vi "Load Values.vi"(11 "Dashboard Data":T1={"Drive PID - Low"={"D"=0.0, "F"=0.0, "RR"=0.0, "IZ"=0.0, "P"=0.0, "I"=0.0}, "Drive PID - High"={"D"=0.0, "F"=0.0, "RR"=0.0, "IZ"=0.0, "P"=0.0, "I"=0.0}, "Vision Settings"={"LED Color"={"Hue"={107.81818389892578, 139.81818389892578}, "Sat"={176.07142857142858, 255.0}, "Val"={40.53571428571429, 255.0}}, "Vision Line"=0.0, "Vision Bottom Clip"=0.0}, "Robot Name"="", "Winch Out"=0.0, "Winch In"=0.0, "Shooter Settings"={"Shooter PID"={"D"=0.0, "F"=0.0, "RR"=0.0, "IZ"=0.0, "P"=0.0, "I"=0.0}, "Instake Belt PID"={"D"=0.0, "F"=0.0, "RR"=0.0, "IZ"=0.0, "P"=0.0, "I"=0.0}, "Shooter Wheel RPM"=0.0, "Instake Belt RPM"=0.0, "Grinder Power"=0.0, "Ramp Up Speed"=0.0}} {"Vision Settings"."LED Color"."Hue" scale=0.0..255.0 scale format="%#_3g"}) -> ()   [LabVIEW 2016]
uses:
  Dashboard Data.ctl
  PID Settings.ctl
  Vision Data.ctl
  Shooter Settings.ctl
  <vilib>/Rock Robotics/WPI/Solenoid/WPI_SolenoidValue.ctl
  <vilib>/Rock Robotics/WPI/Utilities/WPI_GetSetVariantRefNum.vi
  2017 Robot Project/Ball Shooter/Implementation/Ball Shooter Global.vi
  2017 Robot Project/Winch/Implementation/Winch Globals.vi
  <vilib>/Rock Robotics/WPI/Solenoid/WPI_SolenoidSetEnum.vi
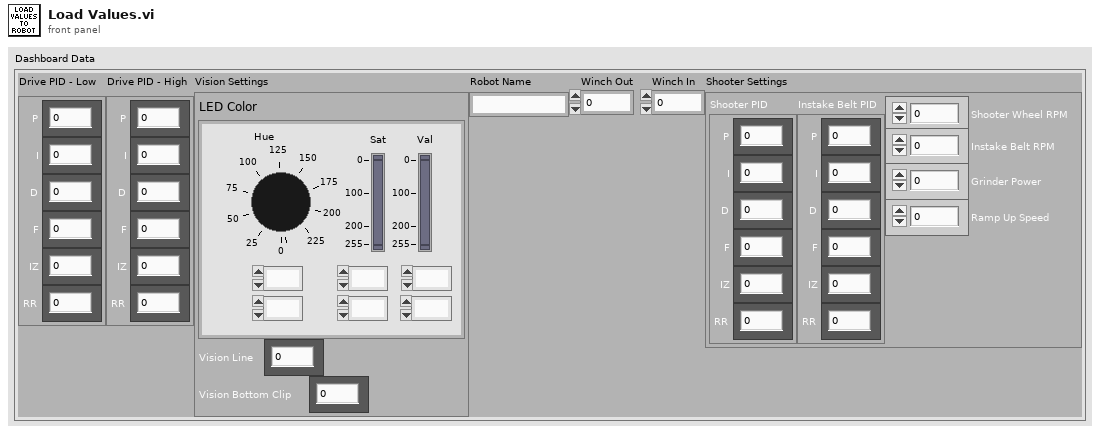
[diagram p1: front panel]
types:
  T1 = typedef "Dashboard Data.ctl" = cluster{"Drive PID - Low":T2, "Drive PID - High":T2, "Vision Settings":T3, "Robot Name":string, "Winch Out":dbl, "Winch In":dbl, "Shooter Settings":T4}
  T2 = typedef "PID Settings.ctl" = cluster{"D":dbl, "F":dbl, "RR":dbl, "IZ":dbl, "P":dbl, "I":dbl}
  T3 = typedef "Vision Data.ctl" = cluster{"LED Color":cluster{"Hue":cluster{dbl, dbl}, "Sat":cluster{dbl, dbl}, "Val":cluster{dbl, dbl}}, "Vision Line":dbl, "Vision Bottom Clip":dbl}
  T4 = typedef "Shooter Settings.ctl" = cluster{"Shooter PID":T2, "Instake Belt PID":T2, "Shooter Wheel RPM":dbl, "Instake Belt RPM":dbl, "Grinder Power":dbl, "Ramp Up Speed":dbl}
  T5 = typedef "WPI_SolenoidValue.ctl" = enum16{"Off", "On", "Forward", "Reverse"}
  T6 = typedef "WPI_RobotDriveDevRef.ctl" = cluster{"DevStatus":errorcluster, "Motors[]":T7[], "Square Inputs":bool, "Max Output":dbl}
  T7 = typedef "WPI_MotorControlDeviceRef.ctl" = cluster{"DeviceStatus":errorcluster, "Type":T8, "PWM":cluster{"PWM Channel":T9, "DeadBand":T10}, "CAN":cluster{"Device Number":u8, "SetOutput VI Ref":variant, "GetOutput VI Ref":variant, "Enable VI Ref":variant, "Disable VI Ref":variant, "Data":variant}, "Invert":bool}
  T8 = typedef "WPI_MotorControlType.ctl" = enum16{"PWM", "CAN"}
  T9 = typedef "FPGA_DIOPWMChannel.ctl" = enum8{"PWM 0", "PWM 1", "PWM 2", "PWM 3", "PWM 4", "PWM 5", "PWM 6", "PWM 7", "PWM 8", "PWM 9", "PWM MXP 0", "PWM MXP 1", "PWM MXP 2", "PWM MXP 3", "PWM MXP 4", "PWM MXP 5", "PWM MXP 6", "PWM MXP 7", "PWM MXP 8", "PWM MXP 9", "Invalid"}
  T10 = typedef "WPI_PWMDeadband.ctl" = cluster{"Name":string, "maxPositivePwm":i32, "minPositivePwm":i32, "centerPwm":i32, "maxNegativePwm":i32, "minNegativePwm":i32, "angularRange":u16}
  T11 = typedef "WPI_SolenoidDevRef.ctl" = cluster{"DevStatus":errorcluster, "Pneumatics Control Module":u8, "Forward Solenoid Channel":T12, "Reverse Solenoid Channel":T12}
  T12 = typedef "WPI_SolenoidChannel.ctl" = enum8{"Solenoid 0", "Solenoid 1", "Solenoid 2", "Solenoid 3", "Solenoid 4", "Solenoid 5", "Solenoid 6", "Solenoid 7", "Invalid"}
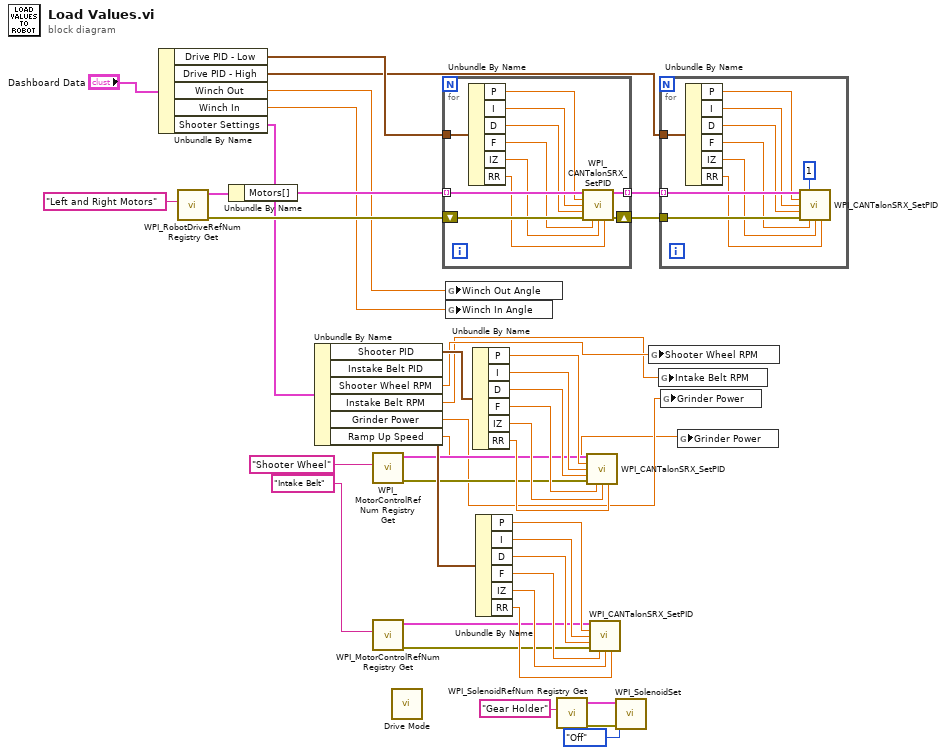
[diagram p0: block diagram]
diagram:
  n1 = Unbundle By Name("Dashboard Data") -> ("Drive PID - Low"=w33:T2, "Drive PID - High"=w32:T2, "Winch Out"=w31:dbl, "Winch In"=w30:dbl, "Shooter Settings"=w23:T4)
  n2 = call <vilib>:"WPI_RobotDriveRefNum Registry Get.vi"("refnum name"="Left and Right Motors") -> ("error out"=w37:errorcluster, "RobotDriveDevRef"=w39:T6)  [unwired: 9 in]
  n3 = Unbundle By Name(w39) -> ("Motors[]"=w38:T7[])
  n4 = Unbundle By Name(w23) -> ("Shooter PID"=w22:T2, "Instake Belt PID"=w15:T2, "Shooter Wheel RPM"=w8:dbl, "Instake Belt RPM"=w7:dbl, "Grinder Power"=w6:dbl, "Ramp Up Speed"=w5:dbl)
  n5 = call <vilib>:"WPI_MotorControlRefNum Registry Get.vi"("refnum name"="Shooter Wheel") -> ("error out"=w12:errorcluster, "MotorControlDevRef"=w13:T7)  [unwired: 9 in]
  n6 = call <vilib>:"WPI_MotorControlRefNum Registry Get.vi"("refnum name"="Intake Belt") -> ("error out"=w10:errorcluster, "MotorControlDevRef"=w11:T7)  [unwired: 9 in]
  n7 = call "Drive Mode.vi"() -> ()  [unwired: 12 in]
  n8 = for {
    tunnel: w38 -> [w50] mode=indexing
    tunnel: w33 -> [w49]
    tunnel: [w42] -> w36 mode=indexing
    shift-right: [w41] -> w35
    shift-left: w37 -> [w51]
    n9 = Unbundle By Name(w49) -> ("P"=w48:dbl, "I"=w47:dbl, "D"=w46:dbl, "F"=w45:dbl, "IZ"=w44:dbl, "RR"=w43:dbl)
    n10 = call <vilib>:"WPI_CANTalonSRX_SetPID.vi"("CAN Talon SRX Ref"=w50, "P"=w48, "I"=w47, "D"=w46, "error in (no error)"=w51, "F"=w45, "I Zone"=w44, "Ramp Rate"=w43) -> ("CAN Talon SRX Ref"=w42:T7, "error out"=w41:errorcluster)  [unwired: 6 in]
  }
  n11 = global write "Winch Globals.vi" "Winch Out Angle"(w31) -> ()
  n12 = global write "Winch Globals.vi" "Winch In Angle"(w30) -> ()
  n13 = Unbundle By Name(w22) -> ("P"=w25:dbl, "I"=w26:dbl, "D"=w27:dbl, "F"=w28:dbl, "IZ"=w29:dbl, "RR"=w24:dbl)
  n14 = Unbundle By Name(w15) -> ("P"=w20:dbl, "I"=w19:dbl, "D"=w18:dbl, "F"=w17:dbl, "IZ"=w16:dbl, "RR"=w21:dbl)
  n15 = call <vilib>:"WPI_SolenoidRefNum Registry Get.vi"("refnum name"="Gear Holder") -> ("error out"=w2:errorcluster, "SolenoidDevRef"=w3:T11)  [unwired: 9 in]
  n16 = call <vilib>:"WPI_CANTalonSRX_SetPID.vi"("CAN Talon SRX Ref"=w13, "P"=w25, "I"=w26, "D"=w27, "error in (no error)"=w12, "F"=w28, "I Zone"=w29, "Ramp Rate"=w24) -> ()  [unwired: 6 in, 2 out]
  n17 = call <vilib>:"WPI_CANTalonSRX_SetPID.vi"("CAN Talon SRX Ref"=w11, "P"=w20, "I"=w19, "D"=w18, "error in (no error)"=w10, "F"=w17, "I Zone"=w16, "Ramp Rate"=w21) -> ()  [unwired: 6 in, 2 out]
  n18 = call-poly <vilib>:"WPI_SolenoidSet.vi"("error in (no error)"=w2, "Value"=WPI_SolenoidValue."Off", "SolenoidDevRef"=w3) -> ()  [unwired: 7 in, 2 out]
  n19 = global write "Ball Shooter Global.vi" "Shooter Wheel RPM"(w8) -> ()
  n20 = global write "Ball Shooter Global.vi" "Intake Belt RPM"(w7) -> ()
  n21 = for {
    tunnel: w36 -> [w60] mode=indexing
    tunnel: w35 -> [w61]
    tunnel: w32 -> [w59]
    n22 = Unbundle By Name(w59) -> ("P"=w58:dbl, "I"=w57:dbl, "D"=w56:dbl, "F"=w55:dbl, "IZ"=w54:dbl, "RR"=w53:dbl)
    n23 = call <vilib>:"WPI_CANTalonSRX_SetPID.vi"("CAN Talon SRX Ref"=w60, "Parameter Slot"=u8 1, "P"=w58, "I"=w57, "D"=w56, "error in (no error)"=w61, "F"=w55, "I Zone"=w54, "Ramp Rate"=w53) -> ()  [unwired: 5 in, 2 out]
  }
  n24 = global write "Ball Shooter Global.vi" "Grinder Power"(w6) -> ()
  n25 = global write "Ball Shooter Global.vi" "Grinder Power"(w5) -> ()
